vi "Sort Aliases.vi"(8 "error in (no error)":errorcluster, 9 "Descending":bool, 10 "index":u32, 11 "Aliases":T1[](array[typedef])) -> (0 "error out":errorcluster, 3 "Sorted Aliases":T1[](array[typedef]))   [LabVIEW 2019, in "Routing and Faulting System Explorer.lvlib"]
uses:
  Routing and Faulting System Explorer.lvlib
  Alias.ctl
  Endpoint.ctl
  81225eb6-56ec-4ce0-96a6-be930ac36616.vi
  81225eb6-56ec-4ce0-96a6-be930ac36616.vi/10c722d5-6e57-4282-9987-57b8967897d4.vi
  81225eb6-56ec-4ce0-96a6-be930ac36616.vi/b6dbaf7c-0239-4974-98db-cadfaeb3d778.vi
  Shared/UI Common/Natural String Merge Sort.vi
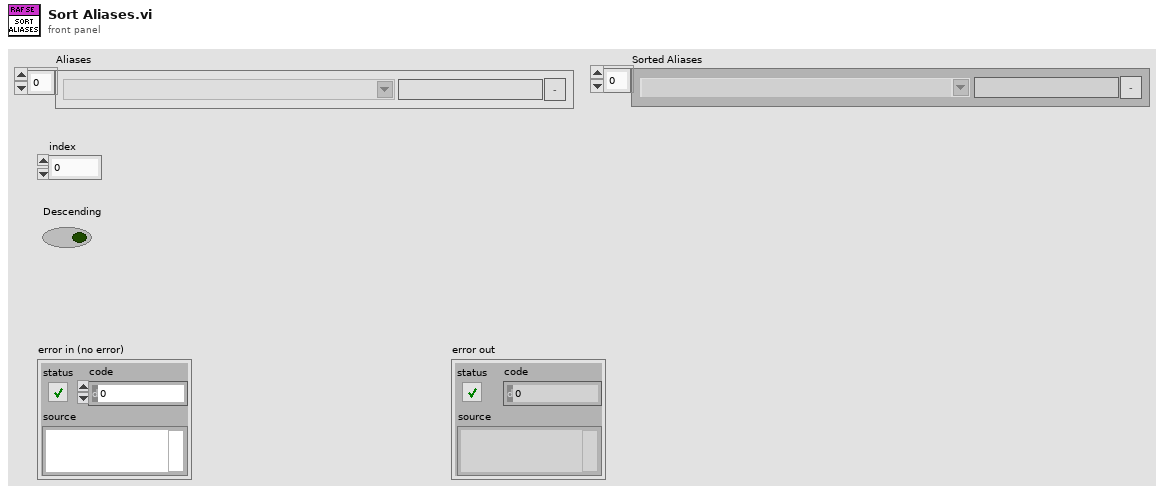
[diagram p1: front panel]
types:
  T1 = typedef "Routing and Faulting System Explorer.lvlib/Alias.ctl" = cluster{"Endpoint":T2, "Alias":string, "Remove":bool}
  T2 = typedef "Routing and Faulting System Explorer.lvlib/Endpoint.ctl" = string
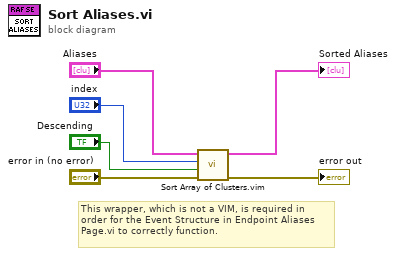
[diagram p0: block diagram]
diagram:
  # "This wrapper, which is not a VIM, is required in\norder for the Event Structure in Endpoint Aliases\nPage.vi to correctly function."
  n1 = call "Sort Array of Clusters.vim"("error in (no error)"="error in (no error)", "Descending"="Descending", "index"="index", "Array"="Aliases") -> ("error out"=→"error out":errorcluster, "Sorted Array"=→"Sorted Aliases":T1[])  [unwired: 6 in]
